vi "Set Cell Color.vi"(6 "Color.lvclass":refnum<class "Color.lvclass">, 8 "error in (no error)":errorcluster, 9 "rowIndex":i32, 10 "colindex":i32, 11 "DataGridView in":refnum<class "DataGridView.lvclass">) -> (0 "error out":errorcluster, 3 "DataGridView out":refnum<class "DataGridView.lvclass">)   [LabVIEW 2013, in "DataGrid.lvlib" / "DataGridView.lvclass"]
doc: "Sets the cell color for one of four cell properties: FG, BK, SelectionFG, SelectionBK. Requires the Color class input, that is used to generate colors from names or RGB values.\n\nThis operation if done on MANY cells iteratively, its best to hide the grid and show it when complete on initialitization for speed."
uses:
  DataGridView.lvclass
  Color/Color.lvclass
  DataGridView.lvclass/DataGridView.ctl
  System.Windows.Forms
  Properties/Read DataGridView.vi
  System.Drawing
panel:
  in  "Property":T1(ring)
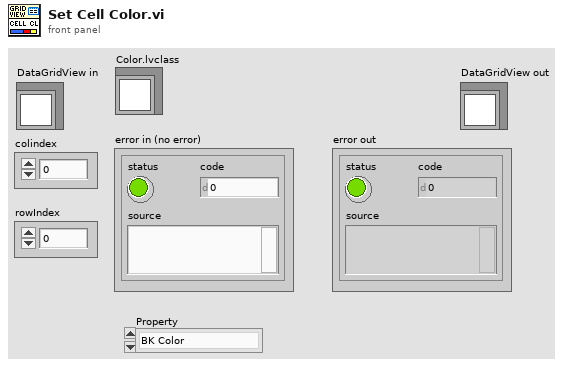
[diagram p1: front panel]
types:
  T1 = enum16{"BK Color", "FG Color", "Selection BK Color", "Selection FG Color"}
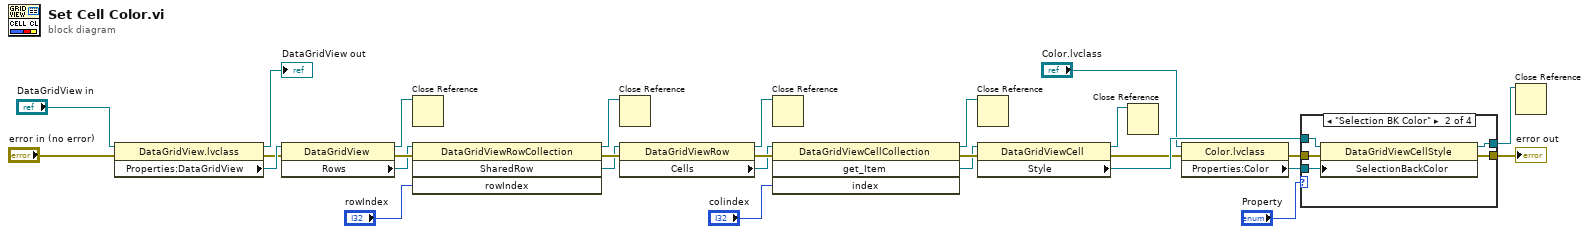
[diagram p0: block diagram]
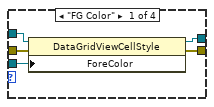
[diagram p2: hidden frame]
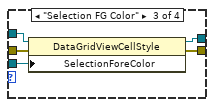
[diagram p3: hidden frame]
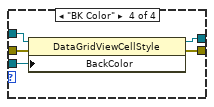
[diagram p4: hidden frame]
diagram:
  n1 = property class="DataGridView.lvclass"(reference="DataGridView in", error in="error in (no error)") -> (reference out=→"DataGridView out":refnum<class "DataGridView.lvclass">, error out=w11:errorcluster, "Properties:DataGridView"=w12:refnum<k24>)
  n2 = property class="DataGridView"(reference=w12, error in=w11) -> (reference out=w9:refnum<k24>, error out=w20:errorcluster, "Rows"=w13:refnum<k24>)
  n3 = Close Reference(reference=w9) -> ()  [unwired: 1 in, 1 out]
  n4 = invoke class="DataGridViewRowCollection" method="SharedRow"(reference=w13, error in=w20, "rowIndex"="rowIndex") -> (reference out=w24:refnum<k24>, error out=w21:errorcluster, "SharedRow"=w14:refnum<k24>)  [unwired: 1 in, 1 out]
  n5 = Close Reference(reference=w24) -> ()  [unwired: 1 in, 1 out]
  n6 = property class="DataGridViewRow"(reference=w14, error in=w21) -> (reference out=w25:refnum<k24>, error out=w22:errorcluster, "Cells"=w15:refnum<k24>)
  n7 = Close Reference(reference=w25) -> ()  [unwired: 1 in, 1 out]
  n8 = invoke class="DataGridViewCellCollection" method="get_Item"(reference=w15, error in=w22, "index"="colindex") -> (reference out=w26:refnum<k24>, error out=w23:errorcluster, "get_Item"=w17:refnum<k24>)  [unwired: 1 in, 1 out]
  n9 = Close Reference(reference=w26) -> ()  [unwired: 1 in, 1 out]
  n10 = property class="DataGridViewCell"(reference=w17, error in=w23) -> (reference out=w27:refnum<k24>, error out=w3:errorcluster, "Style"=w18:refnum<k24>)
  n11 = Close Reference(reference=w27) -> ()  [unwired: 1 in, 1 out]
  n12 = property class="Color.lvclass"(reference="Color.lvclass", error in=w3) -> (error out=w2:errorcluster, "Properties:Color"=w1:refnum<k24>)  [unwired: 1 out]
  n13 = case shown="\"Selection BK Color\"" "Property" {
    tunnel: [w33 w38 w43 w48] -> w28
    tunnel: w2 -> [w32 w37 w42 w44]
    tunnel: w18 -> [w31 w36 w41 w47]
    tunnel: [w30 w35 w40 w46] -> w7
    tunnel: w1 -> [w29 w34 w39 w45]
    frame "FG Color" {
      n14 = property class="DataGridViewCellStyle"(reference=w31, error in=w32, "ForeColor"=w29) -> (reference out=w33:refnum<k24>, error out=w30:errorcluster)
    }
    frame "Selection BK Color" {
      n15 = property class="DataGridViewCellStyle"(reference=w36, error in=w37, "SelectionBackColor"=w34) -> (reference out=w38:refnum<k24>, error out=w35:errorcluster)
    }
    frame "Selection FG Color" {
      n16 = property class="DataGridViewCellStyle"(reference=w41, error in=w42, "SelectionForeColor"=w39) -> (reference out=w43:refnum<k24>, error out=w40:errorcluster)
    }
    frame "BK Color" {
      n17 = property class="DataGridViewCellStyle"(reference=w47, error in=w44, "BackColor"=w45) -> (reference out=w48:refnum<k24>, error out=w46:errorcluster)
    }
  }
  "error out" <- w7
  n18 = Close Reference(reference=w28) -> ()  [unwired: 1 in, 1 out]
